vi "TCP-Receive String (bytes).vi"(0 "connection ID":refnum<k5>, 9 "timeout (ms)":i32=5000, 11 "error in (no error)":errorcluster) -> (4 "connection ID out":refnum<k5>, 8 "data":string, 15 "error out":errorcluster)   [LabVIEW 2020]
panel:
  out "length":i32
  out "unsigned byte array":u8[](array[numeric])
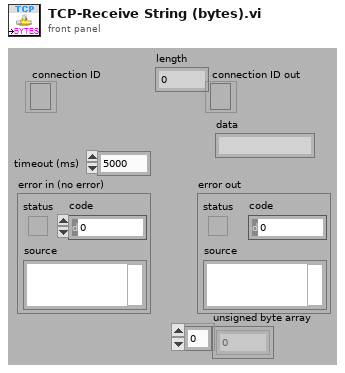
[diagram p1: front panel]
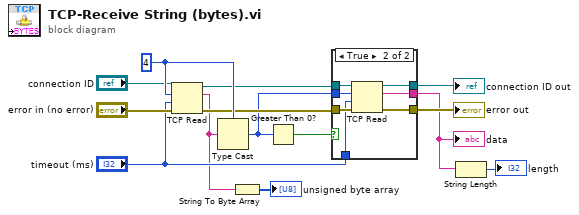
[diagram p0: block diagram]
diagram:
  w14 = 4
  n1 = TCP Read(connection ID="connection ID", bytes to read=w14, error in (no error)="error in (no error)", 9:"timeout (ms)") -> (connection ID out=w11:refnum<k5>, data out=w4:string, error out=w12:errorcluster)  [unwired: 1 in]
  n2 = Type Cast(type=w14, x=w4) -> (*(type *) &x=w9:i32)
  n3 = String To Byte Array(string=w4) -> (unsigned byte array=→"unsigned byte array":u8[])
  n4 = Greater Than 0?(x=w9) -> (x > 0?=w8:bool)
  n5 = case shown="True" w8 {
    tunnel: [_ w23] -> w2
    tunnel: [w16 w22] -> w7
    tunnel: w11 -> [w15 w21]
    tunnel: w12 -> [w16 w20]
    tunnel: w9 -> [_ w19]
    tunnel: [w15 w18] -> w10
    tunnel: "timeout (ms)" -> [_ w17]
    frame False {
    }
    frame True {
      n6 = TCP Read(connection ID=w21, bytes to read=w19, error in (no error)=w20, 9:w17) -> (connection ID out=w18:refnum<k5>, data out=w23:string, error out=w22:errorcluster)  [unwired: 1 in]
    }
  }
  "error out" <- w7
  "data" <- w2
  "connection ID out" <- w10
  n7 = String Length(string=w2) -> (length=→"length":i32)
